vi "GDeviationStatistics.vi"() -> ()   [LabVIEW 2023]
panel:
  in  "X":i64=4
  out "tmp Array":u64[][](array[numeric])
  out "count":i32
  out "MatchArray":u64[](array[numeric])
  out "1D UArr":u64[](array[numeric])
  in  "1D":i64[](array[numeric])
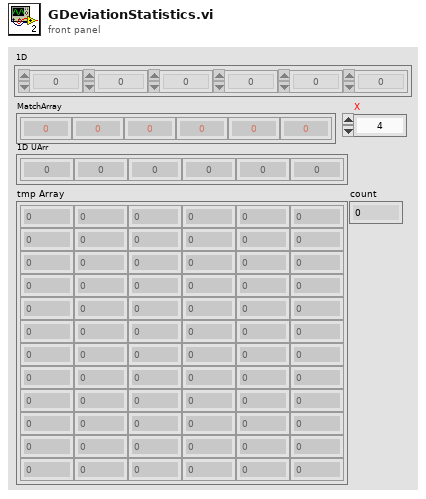
[diagram p1: front panel]
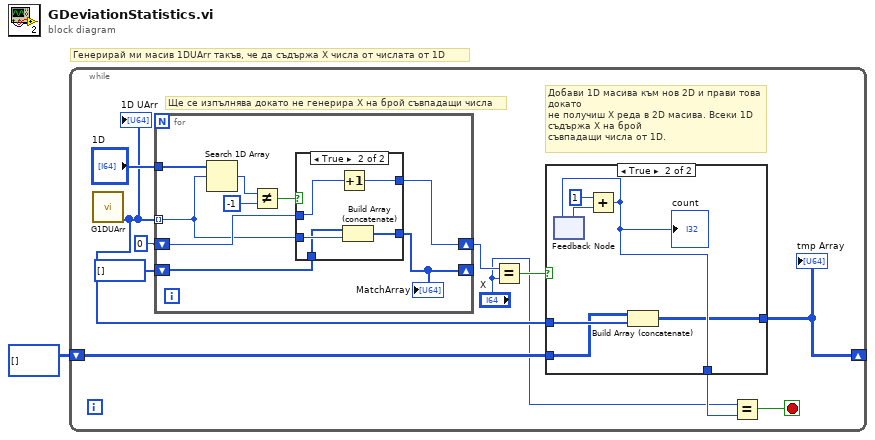
[diagram p0: block diagram]
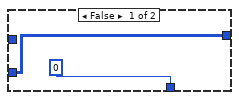
[diagram p2: hidden frame]
diagram:
  # "Генерирай ми масив 1DUArr такъв, че да съдържа Х числа от числата от 1D"
  n1 = while {
    shift-right: [w4] -> _
    shift-left: u64[][] [] -> [w3]
    stop <- w9 stop-if-true
    # "Добави 1D масива към нов 2D и прави това докато\nне получиш X реда в 2D масива. Всеки 1D съдържа Х на брой\nсъвпадащи числа от 1D."
    # "Ще се изпълнява докато не генерира X на брой съвпадащи числа"
    n2 = call "G1DUArr.vi"() -> ("1D UArr"=w5:u64[])  [unwired: 11 in]
    "1D UArr" <- w5
    n3 = for {
      tunnel: w5 -> [w23] mode=indexing
      tunnel: "1D" -> [w29]
      shift-right: [w25] -> w8
      shift-left: i64 0 -> [w24]
      shift-right: [w22] -> _
      shift-left: u64[] [] -> [w21]
      n4 = Search 1D Array(1D array=w29, element=w23) -> (index of element=w28:i32)  [unwired: 1 in]
      n5 = Not Equal?(x=w28, y=-1) -> (x != y?=w26:bool)
      n6 = case shown="True" w26 {
        tunnel: [w31 w35] -> w25
        tunnel: w24 -> [w31 w36]
        tunnel: w23 -> [_ w34]
        tunnel: [w30 w33] -> w22
        tunnel: w21 -> [w30 w32]
        frame False {
        }
        frame True {
          n7 = Increment(x=w36) -> (x+1=w35:i64)
          n8 = Build Array (concatenate)(w32, w34) -> (w33:u64[])
        }
      }
      "MatchArray" <- w22
    }
    n9 = Equal?(x=w8, y="X") -> (x = y?=w10:bool)
    n10 = case shown="True" w10 {
      tunnel: [0 w18] -> w6
      tunnel: w5 -> [_ w17]
      tunnel: [w13 w16] -> w4
      tunnel: w3 -> [w13 w15]
      frame False {
      }
      frame True {
        n11 = feedback #1() -> (w19:i32)  [unwired: 1 in]
        n12 = Add(x=1, y=w19) -> (x+y=w18:i32)
        "count" <- w18
        n13 = feedback-in #1(w18) -> ()
        n14 = Build Array (concatenate)(w15, w17) -> (w16:u64[][])
      }
    }
    "tmp Array" <- w4
    n15 = Equal?(x="X", y=w6) -> (x = y?=w9:bool)
  }
